vi "HatchLimitGet.vi"() -> (3 "Pressed?":bool)   [LabVIEW 2018]
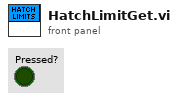
[diagram p1: front panel]
types:
  T1 = typedef "WPI_SwitchDevRef.ctl" = cluster{"DevStatus":errorcluster, "DIO Channel":T2, "CntIndex":T3, "Normally Closed":bool}
  T2 = typedef "FPGA_DIOChannel.ctl" = enum8{"DIO 0", "DIO 1", "DIO 2", "DIO 3", "DIO 4", "DIO 5", "DIO 6", "DIO 7", "DIO 8", "DIO 9", "DIO MXP 0", "DIO MXP 1", "DIO MXP 2", "DIO MXP 3", "DIO MXP 4", "DIO MXP 5", "DIO MXP 6", "DIO MXP 7", "DIO MXP 8", "DIO MXP 9", "DIO MXP 10", "DIO MXP 11", "DIO MXP 12", "DIO MXP 13", "DIO MXP 14", "DIO MXP 15", "SPI Port CS1", "SPI Port CS2", "SPI Port CS3", "SPI Port MISO", "SPI Port MOSI", "Invalid"}
  T3 = typedef "FPGA_CounterCtrSystemIndex.ctl" = enum8{"Ctr 0", "Ctr 1", "Ctr 2", "Ctr 3", "Ctr 4", "Ctr 5", "Ctr 6", "Ctr 7", "Invalid"}
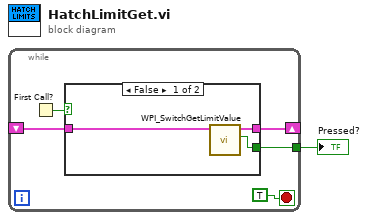
[diagram p0: block diagram]
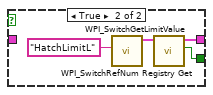
[diagram p2: hidden frame]
diagram:
  n1 = while {
    shift-right: [w4] -> _
    shift-left: _ -> [w2]
    tunnel: [w3] -> w1
    stop <- TRUE stop-if-true
    n2 = First Call?() -> (First Call?: T/F=w5:bool)
    n3 = case shown="False" w5 {
      tunnel: [w8 w11] -> w4
      tunnel: [w7 w10] -> w3
      tunnel: w2 -> [w9 _]
      frame False {
        n4 = call <vilib>:"WPI_SwitchGetLimitValue.vi"("SwitchDevRef"=w9) -> ("Switch Pressed"=w7:bool, "SwitchDevRef"=w8:T1)  [unwired: 8 in, 1 out]
      }
      frame True {
        n5 = call <vilib>:"WPI_SwitchRefNum Registry Get.vi"("refnum name"="HatchLimitL") -> ("SwitchDevRef"=w12:T1)  [unwired: 9 in, 1 out]
        n6 = call <vilib>:"WPI_SwitchGetLimitValue.vi"("SwitchDevRef"=w12) -> ("Switch Pressed"=w10:bool, "SwitchDevRef"=w11:T1)  [unwired: 8 in, 1 out]
      }
    }
  }
  "Pressed?" <- w1
